vi "Cal Rate.vi"(8 "error in (no error)":errorcluster, 11 "Automation in":refnum<class "Automation.lvclass">) -> (0 "error out":errorcluster, 1 "Latest Rate":dbl, 2 "mean Rate":dbl format="%.9f", 3 "Automation out":refnum<class "Automation.lvclass">)   [LabVIEW 2019, in "Automation.lvclass"]
uses:
  Automation.lvclass
  Automation.lvclass/Automation.ctl
  <vilib>/Analysis/baseanly.llb/Mean (DBL).vi
  <vilib>/Analysis/NI_AALBase.lvlib
panel:
  out "Slopes":dbl[](array[numeric])
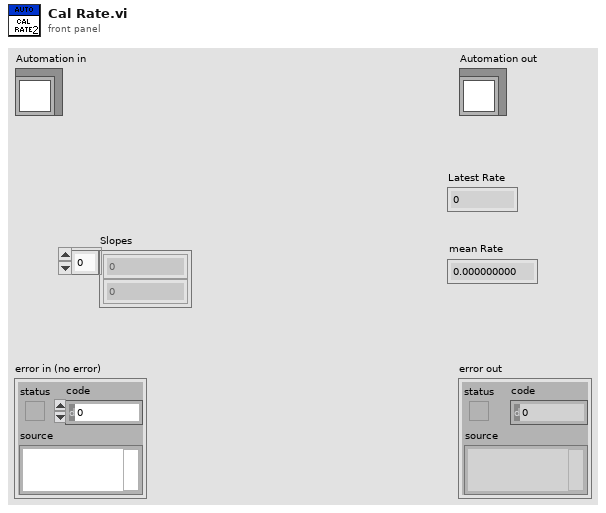
[diagram p1: front panel]
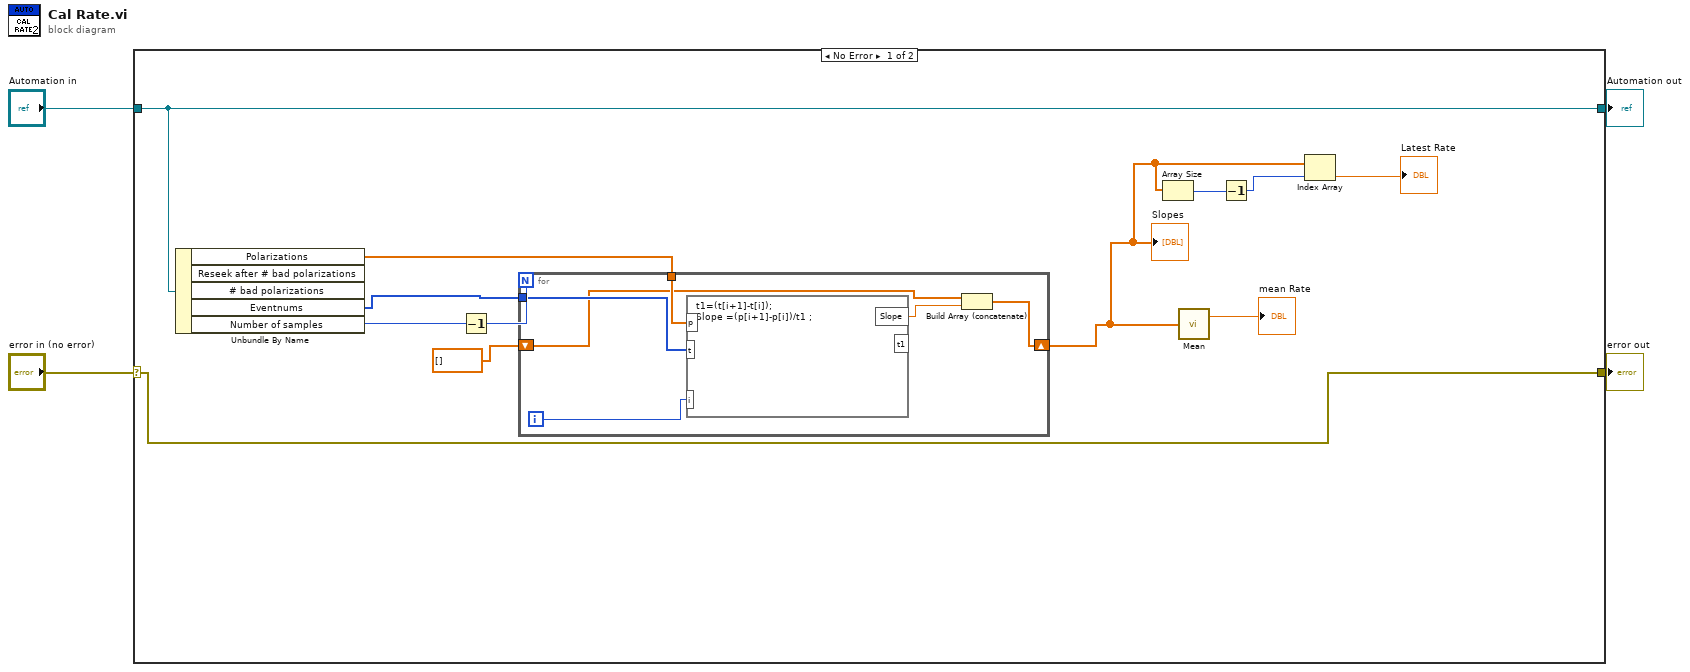
[diagram p0: block diagram]
diagram:
  n1 = case shown="No Error" "error in (no error)" {
    selector: "error in (no error)" -> [w9 w24]
    tunnel: [w14 w23] -> w2
    tunnel: "Automation in" -> [w14 w23]
    tunnel: [w9 w24] -> w1
    frame No Error {
      n2 = Unbundle By Name(w14) -> ("Polarizations"=w10:dbl[], "Eventnums"=w12:i64[], "Number of samples"=w13:i32)  [unwired: 2 out]
      n3 = Decrement(x=w13) -> (x-1=w16:i32)
      n4 = for {
        N: w16 -> [_]
        tunnel: w10 -> [w22]
        tunnel: w12 -> [w21]
        shift-right: [w17] -> w8
        shift-left: dbl[] [] ("appended array") -> [w18]
        i -> [w20]
        n5 = formula code="t1=(t[i+1]-t[i]);\nSlope =(p[i+1]-p[i])/t1 ;"("p"=w22, "t"=w21, "i"=w20) -> ("Slope"=w19:dbl)  [unwired: 1 out]
        n6 = Build Array (concatenate)(w18, w19) -> (w17:dbl[])
      }
      "Slopes" <- w8
      n7 = Array Size(array=w8) -> (size(s)=w7:i32)
      n8 = call-poly <vilib>:"Mean.vi"("X"=w8) -> ("mean"=→"mean Rate":dbl)  [unwired: 1 out]
      n9 = Decrement(x=w7) -> (x-1=w6:i32)
      n10 = Index Array(array=w8, index=w6) -> (element=→"Latest Rate":dbl)
    }
    frame Error {
    }
  }
  "error out" <- w1
  "Automation out" <- w2
